vi "WaveGenerator.vi"(5 "TestLoops":i32, 6 "AxisForce":dbl[](array[numeric]), 7 "dt":dbl, 8 "Angle":dbl[](array[numeric]), 9 "WaveDefineArray":T1[](array[typedef]) {"Enable" items=["不使能", "使能"]; "Wave" items=["0指令", "正弦波", "方波", "三角波", "常值", "波形数据", "白噪声", "正弦扫频", "梯度加载", "VMIC"]; "ChannelType" items=["标准波形跟踪"=1, "扫频测试"=2, "消除多余力"=3, "梯度加载"=4, "载荷谱跟踪"=5, "模拟输入跟踪"=9]; "ChannelStatus" items=["通道关", "位置通道", "加载通道"]}, 10 "VMIC command":dbl[](array[numeric]), 11 "Data array":dbl[][](array[numeric])) -> (0 "type out":dbl[](array[numeric]), 1 "Boolean":bool, 2 "Command":dbl[](array[numeric]), 3 "wave out 2":dbl[](array[numeric]))   [LabVIEW 2014]
uses:
  ChannelCommand.ctl
  Control 1.ctl
  WaveType.ctl
  MoterEnable.ctl
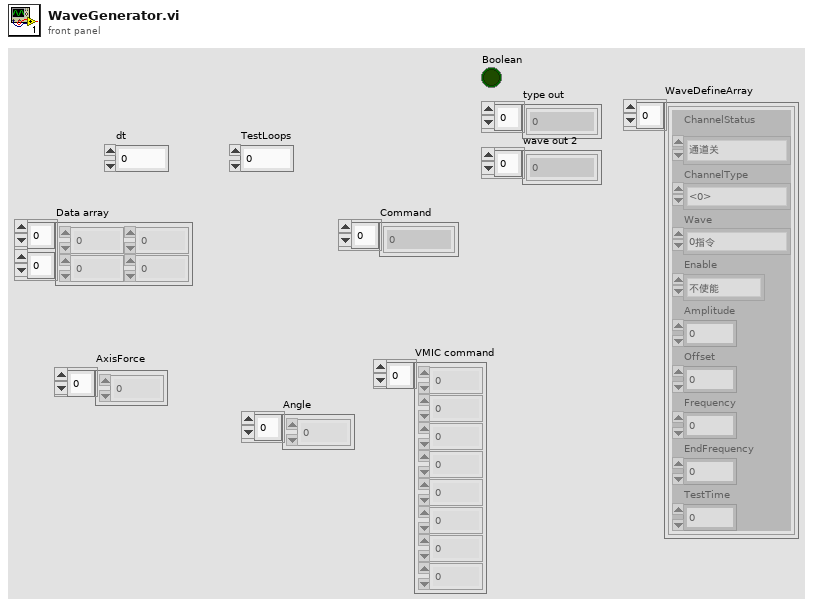
[diagram p1: front panel]
types:
  T1 = typedef "ChannelCommand.ctl" = cluster{"ChannelStatus":T2, "ChannelType":i32, "Wave":T3, "Enable":T4, "Amplitude":dbl, "Offset":dbl, "Frequency":dbl, "EndFrequency":dbl, "TestTime":dbl}
  T2 = typedef "Control 1.ctl" = i32
  T3 = typedef "WaveType.ctl" = i32
  T4 = typedef "MoterEnable.ctl" = u16
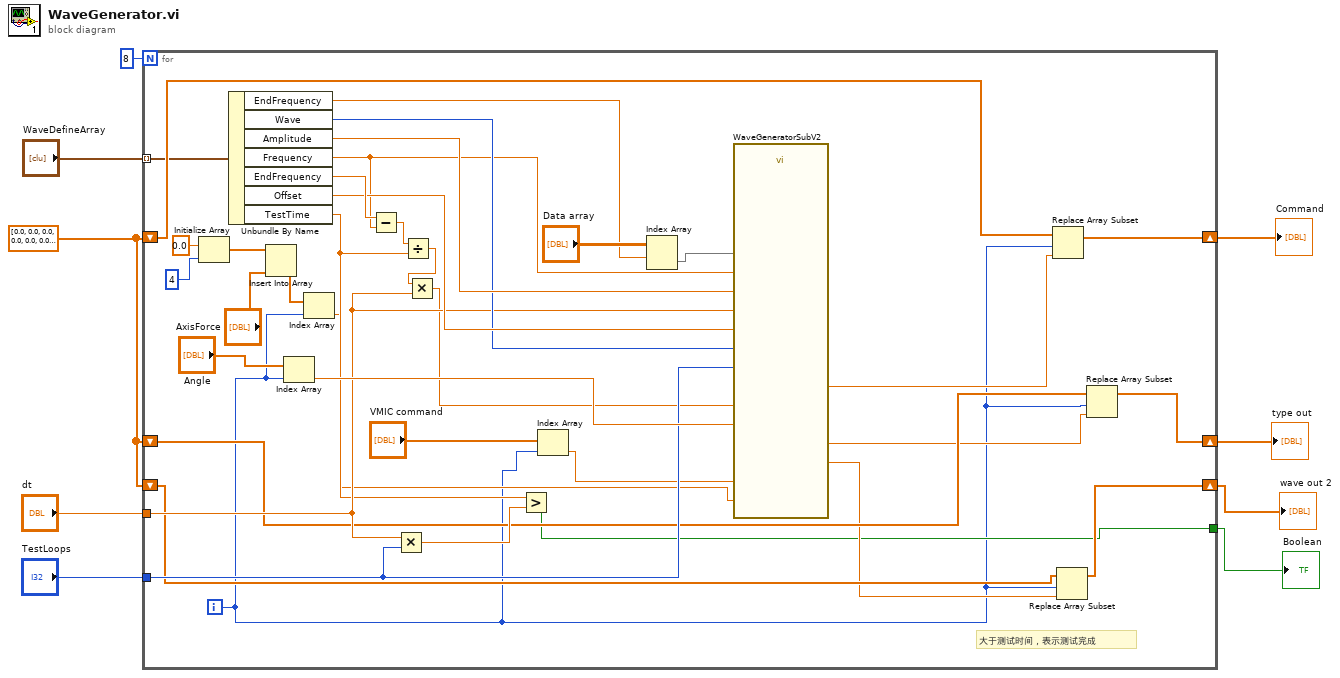
[diagram p0: block diagram]
diagram:
  w3 = dbl[] [0.0, 0.0, 0.0, 0.0, 0.0, 0.0, 0.0, 0.0]
  n1 = for {
    N: 8 -> [_]
    tunnel: "dt" -> [w30]
    tunnel: "TestLoops" -> [w31]
    tunnel: "WaveDefineArray" -> [w44] mode=indexing
    shift-right: [w45] -> w6
    shift-left: w3 -> [w46]
    tunnel: [w12] -> w2
    shift-right: [w26] -> w5
    shift-left: w3 -> [w25]
    shift-right: [w23] -> w4
    shift-left: w3 -> [w22]
    i -> [w10]
    # "大于测试时间，表示测试完成"
    n2 = Initialize Array(0.0 ("元素"), 4 ("维数大小")) -> (w14:dbl[])
    n3 = Unbundle By Name(w44) -> ("EndFrequency"=w42:dbl, "Wave"=w35:T3, "Amplitude"=w37:dbl, "Frequency"=w28:dbl, "EndFrequency"=w41:dbl, "Offset"=w36:dbl, "TestTime"=w27:dbl)
    n4 = Insert Into Array(array=w14, new element="AxisForce") -> (w13:dbl[])  [unwired: 1 in]
    n5 = Index Array(array="Angle", index=w10) -> (element=w33:dbl)
    n6 = Index Array(array=w13, index=w10) -> (element=w11:dbl)
    n7 = Subtract(x=w41, y=w28) -> (x-y=w40:dbl)
    n8 = Multiply(x=w30, y=w31) -> (x*y=w29:dbl)
    n9 = Divide(x=w40, y=w27) -> (x/y=w39:dbl)
    n10 = Multiply(x=w39, y=w30) -> (x*y=w18:dbl)
    n11 = Greater?(x=w27, y=w29) -> (0:w12:bool)
    n12 = Index Array(array="VMIC command", index=w10) -> (element=w19:dbl)
    n13 = Index Array(array="Data array", index (row)=w42) -> (element=w38:dbl[])  [unwired: 1 in]
    n14 = call "WaveGeneratorSubV2.vi"("Amplitude"=w37, "Wave"=w35, "ForceSample"=w11, "Data array"=w38, "Frequent"=w28, "Angle"=w33, "Offset"=w36, "deltaF"=w18, "VMIC"=w19, "dt"=w30, "TestLoops"=w31) -> ("Output"=w32:dbl, "Output 2"=w24:dbl, "waveout 3"=w21:dbl)  [unwired: 2 in]
    n15 = Replace Array Subset "Replace Array Subset"(array=w46, new element=w32, index=w10) -> (w45:dbl[])
    n16 = Replace Array Subset "Replace Array Subset"(array=w22, new element=w21, index=w10) -> (w23:dbl[])
    n17 = Replace Array Subset "Replace Array Subset"(array=w25, new element=w24, index=w10) -> (w26:dbl[])
  }
  "Command" <- w6
  "Boolean" <- w2
  "type out" <- w5
  "wave out 2" <- w4
